vi "For tests.vi"() -> ()   [LabVIEW 2017]
uses:
  <instrlib>/Roboteq Controller KBL1xxx/Roboteq Controller KBL1xxx.lvlib
panel:
  out "Sent Command":string
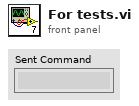
[diagram p1: front panel]
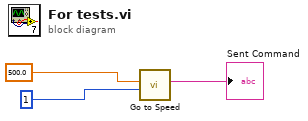
[diagram p0: block diagram]
diagram:
  n1 = call <instrlib>:"Go to Speed.vi"("Channel"=u8 1, "Speed, RPM"=500.0) -> ("Sent Command"=→"Sent Command":string)  [unwired: 7 in, 2 out]
